vi "Data Graph.vi"() -> ()   [LabVIEW 2014]
panel:
  in  "Setup":bool
  out "XY Graph":cluster{"X":dbl, "Y":dbl}[](graph)
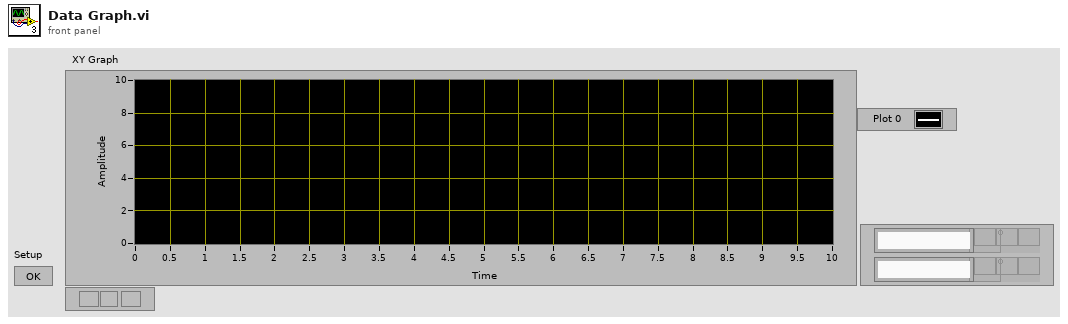
[diagram p1: front panel]
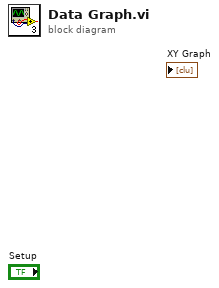
[diagram p0: block diagram]
diagram:
